vi "Splash Screen.vi"() -> ()   [LabVIEW 2015, in "Application Launcher.lvlib"]
doc: "这是应用程序的顶层VI。该VI和许多应用程序的初始屏幕一样， 当应用程序载入内存时吸引用户注意。本应用程序很小，启动时间很短，因此初始屏幕只会瞬间闪烁一下。这种闪烁看上去不舒服，因此本VI添加了一个三秒钟的延迟，使初始屏幕稍作驻留。\n\n本VI通过调用一个延迟加载的子VI，载入应用程序的其他部分。这样做的好处是，不论VI层次结构有多么庞大，初始屏幕都可以立即启动，而且其他VI的加载成为加载进程中的一个完整步骤。"
uses:
  Application Launcher.lvlib
  Air Cooler Application/Air Cooler Application/Load App.vi
  Air Cooler Application/Air Cooler Application/Air Cooler Application.lvclass
panel:
  out "等待指示灯":T1
  out "应用程序名称":string
  out "当前操作：":string
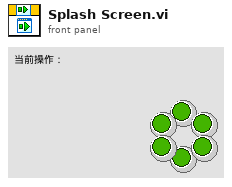
[diagram p1: front panel]
types:
  T1 = cluster{"DNL_wait 1":bool, "DNL_wait 1":bool, "DNL_wait 1":bool, "DNL_wait 1":bool, "DNL_wait 1":bool, "DNL_wait 1":bool}
  T2 = cluster{"[0]":bool, "[1]":bool, "[2]":bool, "[3]":bool, "[4]":bool, "[5]":bool}
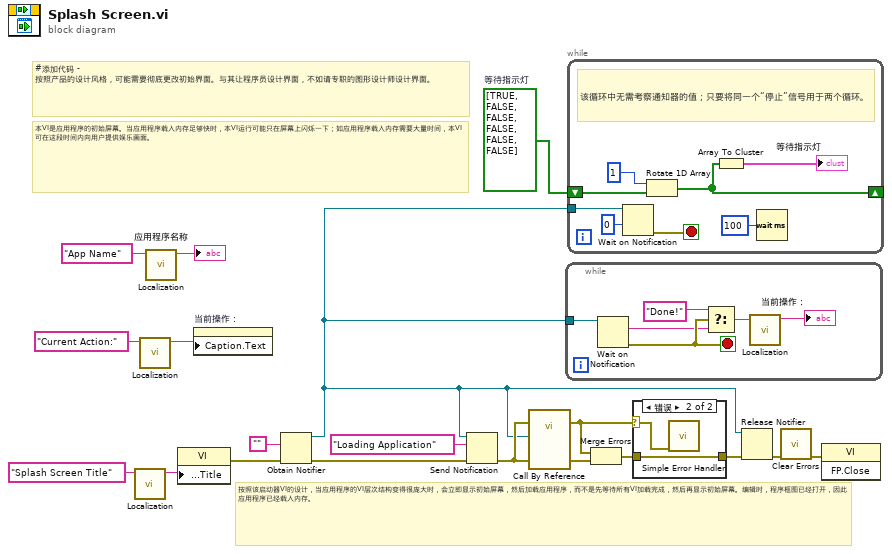
[diagram p0: block diagram]
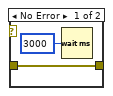
[diagram p2: hidden frame]
diagram:
  w8 = bool[] [TRUE, FALSE, FALSE, FALSE, FALSE, FALSE]  # 等待指示灯
  # "#添加代码 - 按照产品的设计风格，可能需要彻底更改初始界面。与其让程序员设计界面，不如请专职的图形设计师设计界面。"
  # "本VI是应用程序的初始屏幕。当应用程序载入内存足够快时，本VI运行可能只在屏幕上闪烁一下；如应用程序载入内存需要大量时间，本VI可在这段时间内向用户提供娱乐画面。"
  # "按照该启动器VI的设计，当应用程序的VI层次结构变得很庞大时，会立即显示初始屏幕，然后加载应用程序，而不是先等待所有VI加载完成，然后再显示初始屏幕。编辑时，程序框图已经打开，因此应用程序已经载入内存。"
  n1 = call "Localization.vi"("未本地化"="Splash Screen Title" ("Window Title")) -> ("本地化"=w19:string)  [unwired: 10 in]
  n2 = call "Localization.vi"("未本地化"="Current Action:" ("Window Title")) -> ("本地化"=w4:string)  [unwired: 10 in]
  n3 = call "Localization.vi"("未本地化"="App Name" ("Unlocalized")) -> ("本地化"=→"应用程序名称":string)  [unwired: 10 in]
  n4 = property on="Property Node" class="VI"("Front Panel.Title"=w19) -> (error out=w17:errorcluster)  [unwired: 2 in, 1 out]
  n5 = property on="当前操作：" class="Str"("Caption.Text"=w4) -> ()  [unwired: 2 in, 2 out]
  n6 = Obtain Notifier(notification data type="" ("Empty String Constant"), error in (no error)=w17) -> (notifier out=w12:refnum<notifier>, error out=w6:errorcluster)  [unwired: 2 in, 1 out]
  n7 = Send Notification(notification="Loading Application", notifier=w12, error in (no error)=w6) -> (error out=w13:errorcluster)  [unwired: 1 out]
  n8 = call-by-ref "?"(error in=w13, 8:"error in (no error)"=w13, "Status Notifier"=w12) -> (error out=w1:errorcluster, 0:"error out"=w16:errorcluster)  [unwired: 10 in, 1 out]
  n9 = while {
    tunnel: w12 -> [w24]
    stop <- w23 stop-if-true
    n10 = Wait on Notification(notifier=w24) -> (notification=w21:string, error out=w23:errorcluster)  [unwired: 3 in, 2 out]
    n11 = Select(t="Done!" ("notification"), s=w23, f=w21) -> (s? t:f=w20:string)
    n12 = call "Localization.vi"("未本地化"=w20) -> ("本地化"=→"当前操作：":string)  [unwired: 10 in]
  }
  n13 = while {
    shift-right: [w27] -> _
    shift-left: w8 -> [w29]
    tunnel: w12 -> [w31]
    stop <- w33 stop-if-true
    # "该循环中无需考察通知器的值；只要将同一个“停止”信号用于两个循环。"
    n14 = Wait on Notification(notifier=w31, timeout in ms (-1)=0) -> (error out=w33:errorcluster)  [unwired: 2 in, 3 out]
    n15 = Rotate 1D Array(1:w29, 2:1 ("n")) -> (0:w27:bool[])
    n16 = Array To Cluster(array=w27) -> (cluster=→"等待指示灯":T2)
    n17 = Wait (ms)(milliseconds to wait=u32 100) -> ()  [unwired: 1 out]
  }
  n18 = Merge Errors(w1, w16) -> (w2:errorcluster)
  n19 = case shown="错误" w1 {
    tunnel: [w35 w36] -> w3
    tunnel: w2 -> [w35 w36]
    selector: w1 -> [_ w37]
    frame No Error {
      n20 = Wait (ms)(milliseconds to wait=u32 3000) -> ()  [unwired: 1 out]
    }
    frame Error {
      n21 = call <vilib>:"Simple Error Handler.vi"("error in (no error)"=w37) -> ()  [unwired: 4 in, 5 out]
    }
  }
  n22 = Release Notifier(notifier=w12, error in (no error)=w3) -> (error out=w15:errorcluster)  [unwired: 1 in, 2 out]
  n23 = call <vilib>:"Clear Errors.vi"("error in (no error)"=w15) -> ("error out"=w7:errorcluster)  [unwired: 5 in, 1 out]
  n24 = invoke on="Invoke Node" class="VI" method="FP.Close"(error in=w7) -> ()  [unwired: 2 in, 3 out]
